vi "BRig_Host_dataRunState__entryAdd_v4.vi"(0 "input_dataPlot":u16[][](array[numeric]), 1 "input_dataTS":u16[][](array[numeric]), 2 "input_idx":i32[](array[numeric]), 4 "input_nTrial":u16, 5 "input_LorR":u16, 7 "input_sSelection":u16, 8 "input_trig_l2":u16, 9 "input_tSelection":u16, 10 "input_trig_l1":u16, 11 "input_tSelectionPlot":u16, 12 "input_DAB_flipLR":u16, 13 "input_iSelection":u16) -> (14 "output_dataPlot":u16[][](array[numeric]), 15 "output_dataTS":u16[][](array[numeric]), 16 "output_idx":i32[](array[numeric]), 18 "output_updatePlot":bool)   [LabVIEW 2014]
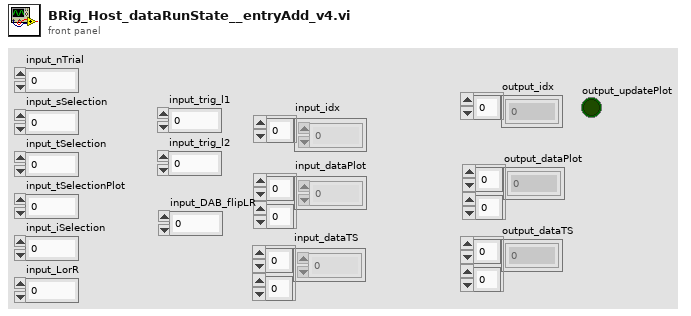
[diagram p1: front panel]
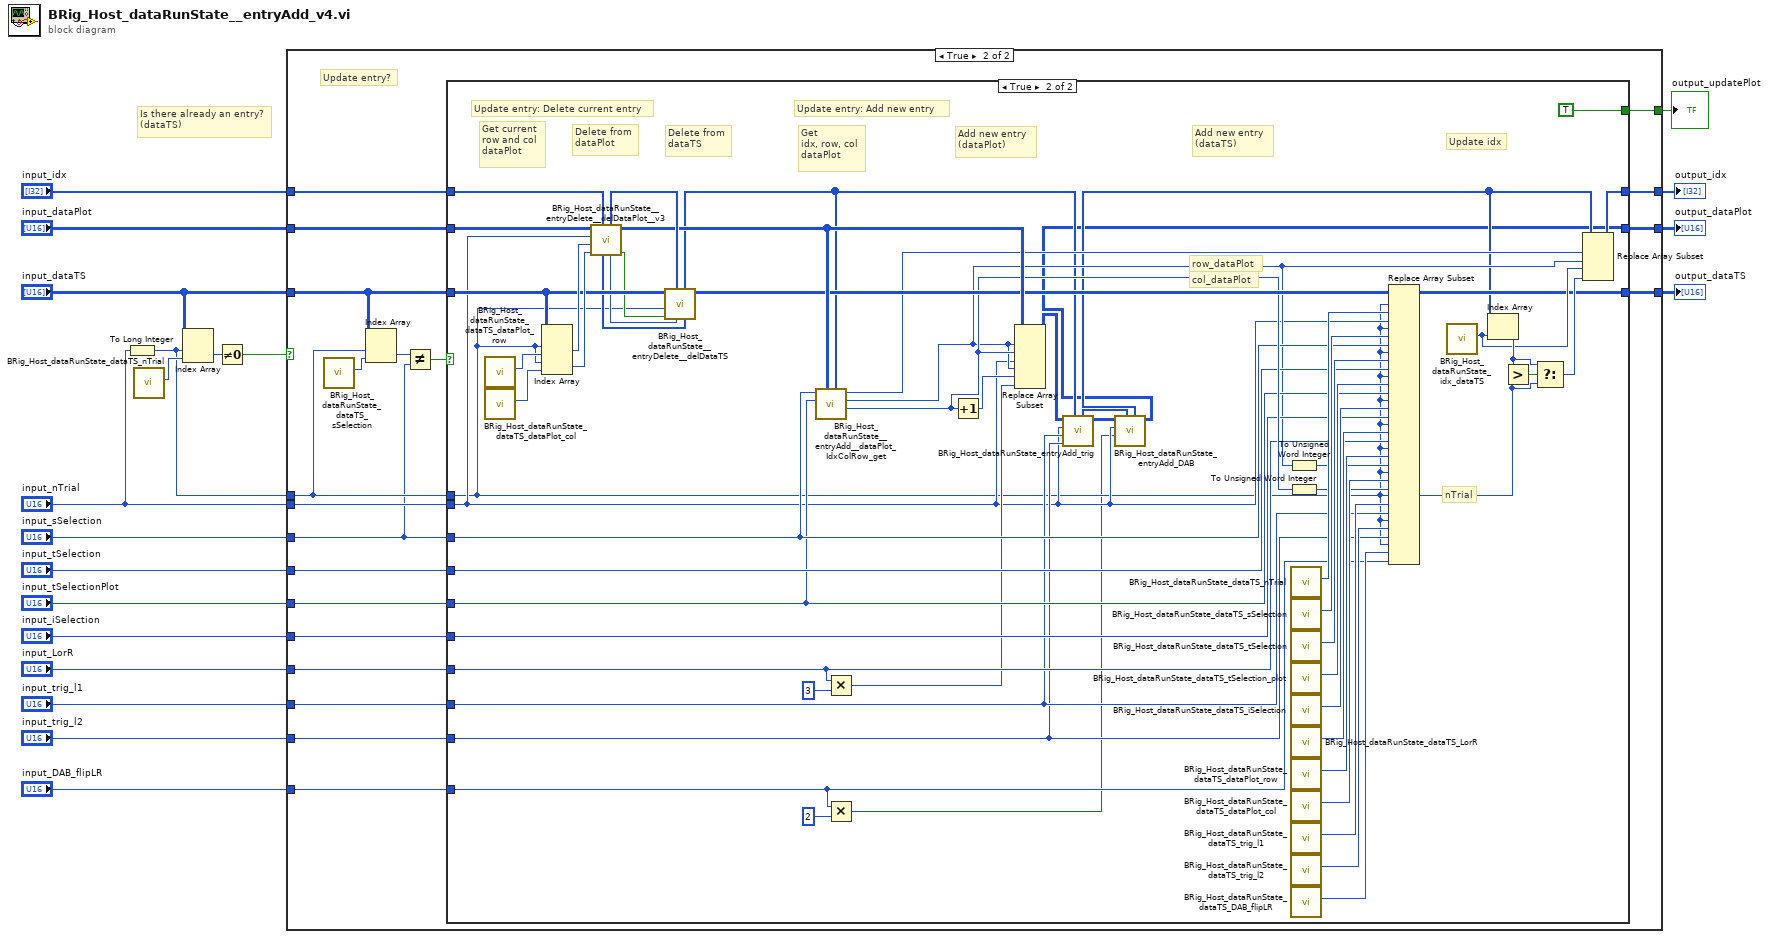
[diagram p0: block diagram]
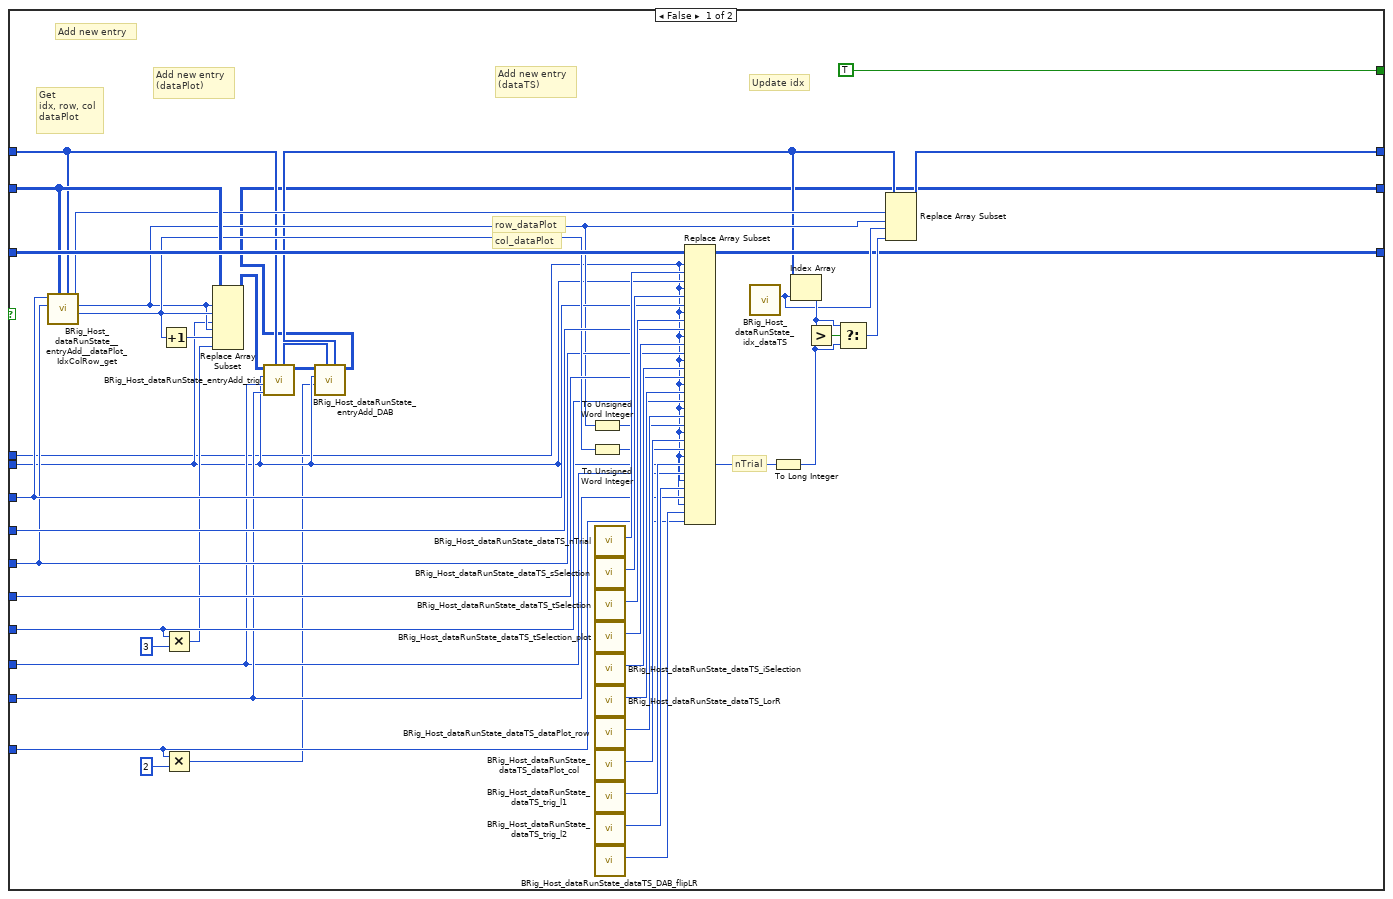
[diagram p2: hidden frame]
diagram:
  # "Is there already an entry?\n(dataTS)"
  n1 = To Long Integer(number="input_nTrial") -> (32bit integer=w16:i32)
  n2 = call "BRig_Host_dataRunState_dataTS_nTrial.vi"() -> ("output_idx_dataTS_nTrial"=w20:i32)  [unwired: 11 in]
  n3 = Index Array(array="input_dataTS", index (row)=w16, index (col)=w20) -> (element=w19:u16)
  n4 = Not Equal To 0?(x=w19) -> (x != 0?=w18:bool)
  n5 = case shown="True" w18 {
    tunnel: "input_nTrial" -> [w26 w77]
    tunnel: w16 -> [w25 w79]
    tunnel: "input_dataTS" -> [w67 w81]
    tunnel: "input_idx" -> [w33 w85]
    tunnel: "input_dataPlot" -> [w45 w83]
    tunnel: "input_sSelection" -> [w42 w71]
    tunnel: "input_tSelectionPlot" -> [w41 w78]
    tunnel: "input_iSelection" -> [w55 w74]
    tunnel: "input_LorR" -> [w36 w76]
    tunnel: [w57 w84] -> w7
    tunnel: [w27 w82] -> w6
    tunnel: [w50 w80] -> w5
    tunnel: "input_tSelection" -> [w56 w75]
    tunnel: [TRUE w73] -> w4
    tunnel: "input_trig_l1" -> [w31 w70]
    tunnel: "input_trig_l2" -> [w32 w69]
    tunnel: "input_DAB_flipLR" -> [w22 w68]
    frame False {
      # "Get\nidx, row, col\ndataPlot"
      # "nTrial"
      # "row_dataPlot"
      # "col_dataPlot"
      # "Update idx"
      # "Add new entry\n(dataPlot)"
      # "Add new entry"
      # "Add new entry\n(dataTS)"
      n6 = call "BRig_Host_dataRunState__entryAdd__dataPlot_IdxColRow_get.vi"("input_idx"=w33, "input_dataPlot"=w45, "input_tSelectionPlot"=w41, "input_sSelection"=w42) -> ("output_col_dataPlot"=w43:i32, "output_row_dataPlot"=w40:i32, "output_idx_dataPlot"=w44:i32)  [unwired: 5 in]
      n7 = Increment(x=w43) -> (x+1=w58:i32)
      n8 = Multiply(x=w36, y=u16 3) -> (x*y=w35:u16)
      n9 = Multiply(x=w22, y=u16 2) -> (x*y=w21:u16)
      n10 = Replace Array Subset(array=w45, new element #1=w26, index (row) #1=w40, index (col) #1=w43, new element #2=w35, index (row) #2=w40, index (col) #2=w58) -> (w34:u16[][])
      n11 = call "BRig_Host_dataRunState_entryAdd_trig.vi"("input_idx"=w33, "input_trig_l2"=w32, "input_trig_l1"=w31, "input_nTrial"=w26, "input_dataPlot"=w34) -> ("output_dataPlot"=w30:u16[][], "output_idx"=w28:i32[])  [unwired: 5 in]
      n12 = call "BRig_Host_dataRunState_entryAdd_DAB.vi"("input_idx"=w28, "input_DAB_flipLR"=w21, "input_nTrial"=w26, "input_dataPlot"=w30) -> ("output_dataPlot"=w27:u16[][], "output_idx"=w29:i32[])  [unwired: 6 in]
      n13 = To Unsigned Word Integer(number=w40) -> (unsigned 16bit integer=w49:u16)
      n14 = To Unsigned Word Integer(number=w43) -> (unsigned 16bit integer=w48:u16)
      n15 = call "BRig_Host_dataRunState_dataTS_nTrial.vi"() -> ("output_idx_dataTS_nTrial"=w66:i32)  [unwired: 11 in]
      n16 = call "BRig_Host_dataRunState_dataTS_sSelection.vi"() -> ("output_idx_dataTS_sSelection"=w65:i32)  [unwired: 11 in]
      n17 = call "BRig_Host_dataRunState_dataTS_tSelection.vi"() -> ("output_idx_dataTS_tSelection"=w64:i32)  [unwired: 11 in]
      n18 = call "BRig_Host_dataRunState_dataTS_tSelection_plot.vi"() -> ("output_idx_dataTS_tSelection_plot"=w63:i32)  [unwired: 11 in]
      n19 = call "BRig_Host_dataRunState_dataTS_iSelection.vi"() -> ("output_idx_dataTS_iSelection"=w62:i32)  [unwired: 11 in]
      n20 = call "BRig_Host_dataRunState_dataTS_LorR.vi"() -> ("output_idx_dataTS_LorR"=w61:i32)  [unwired: 11 in]
      n21 = call "BRig_Host_dataRunState_dataTS_dataPlot_row.vi"() -> ("output_idx_dataTS_dataPlot_row"=w60:i32)  [unwired: 11 in]
      n22 = call "BRig_Host_dataRunState_dataTS_dataPlot_col.vi"() -> ("output_idx_dataTS_dataPlot_col"=w59:i32)  [unwired: 11 in]
      n23 = call "BRig_Host_dataRunState_dataTS_trig_l1.vi"() -> ("output_idx_dataTS_trig_l1"=w38:i32)  [unwired: 11 in]
      n24 = call "BRig_Host_dataRunState_dataTS_trig_l2.vi"() -> ("output_idx_dataTS_trig_l2"=w37:i32)  [unwired: 11 in]
      n25 = call "BRig_Host_dataRunState_dataTS_DAB_flipLR.vi"() -> ("output_idx_dataTS_DAB_flipLR"=w24:i32)  [unwired: 11 in]
      n26 = Replace Array Subset(array=w67, new element #1=w26, index (row) #1=w25, index (col) #1=w66, new element #2=w42, index (row) #2=w25, index (col) #2=w65, new element #3=w56, index (row) #3=w25, index (col) #3=w64, new element #4=w41, index (row) #4=w25, index (col) #4=w63, new element #5=w55, index (row) #5=w25, index (col) #5=w62, new element #6=w36, index (row) #6=w25, index (col) #6=w61, new element #7=w49, index (row) #7=w25, index (col) #7=w60, new element #8=w48, index (row) #8=w25, index (col) #8=w59, new element #9=w31, index (row) #9=w25, index (col) #9=w38, new element #10=w32, index (row) #10=w25, index (col) #10=w37, new element #11=w22, index (row) #11=w25, index (col) #11=w24) -> (w50:u16[][])
      n27 = call "BRig_Host_dataRunState_idx_dataTS.vi"() -> ("output_idx_dataTS"=w52:i32)  [unwired: 11 in]
      n28 = To Long Integer(number=w26) -> (32bit integer=w47:i32)
      n29 = Index Array(array=w29, index=w52) -> (element=w53:i32)
      n30 = Greater?(x=w53, y=w47) -> (0:w54:bool)
      n31 = Select(t=w53, s=w54, f=w47) -> (s? t:f=w51:i32)
      n32 = Replace Array Subset(array=w29, new element #1=w40, index #1=w44, new element #2=w51, index #2=w52) -> (w57:i32[])
    }
    frame True {
      # "Update entry?"
      n33 = call "BRig_Host_dataRunState_dataTS_sSelection.vi"() -> ("output_idx_dataTS_sSelection"=w72:i32)  [unwired: 11 in]
      n34 = Index Array(array=w81, index (row)=w79, index (col)=w72) -> (element=w87:u16)
      n35 = Not Equal?(x=w87, y=w71) -> (x != y?=w86:bool)
      n36 = case shown="True" w86 {
        tunnel: w85 -> [w90 w142]
        tunnel: [w90 w121] -> w84
        tunnel: w83 -> [w89 w145]
        tunnel: [w89 w97] -> w82
        tunnel: w81 -> [w88 w141]
        tunnel: [w88 w118] -> w80
        tunnel: w79 -> [_ w95]
        tunnel: w71 -> [_ w115]
        tunnel: w78 -> [_ w113]
        tunnel: w77 -> [_ w96]
        tunnel: w76 -> [_ w106]
        tunnel: w75 -> [_ w114]
        tunnel: w74 -> [_ w112]
        tunnel: [_ TRUE] -> w73
        tunnel: w70 -> [_ w103]
        tunnel: w69 -> [_ w102]
        tunnel: w68 -> [_ w92]
        frame False {
          # "Do nothing"
        }
        frame True {
          # "nTrial"
          # "row_dataPlot"
          # "col_dataPlot"
          # "Update idx"
          # "Add new entry\n(dataPlot)"
          # "Add new entry\n(dataTS)"
          # "Get\nidx, row, col\ndataPlot"
          # "Update entry: Add new entry"
          # "Delete from\ndataTS"
          # "Delete from\ndataPlot"
          # "Get current\nrow and col\ndataPlot"
          # "Update entry: Delete current entry"
          n37 = call "BRig_Host_dataRunState_dataTS_dataPlot_row.vi"() -> ("output_idx_dataTS_dataPlot_row"=w147:i32)  [unwired: 11 in]
          n38 = call "BRig_Host_dataRunState_dataTS_dataPlot_col.vi"() -> ("output_idx_dataTS_dataPlot_col"=w146:i32)  [unwired: 11 in]
          n39 = Index Array(array=w141, index (row) #1=w95, index (col) #1=w147, index (row) #2=w95, index (col) #2=w146) -> (element #1=w143:u16, element #2=w144:u16)
          n40 = call "BRig_Host_dataRunState__entryDelete__delDataPlot__v3.vi"("input_idx"=w142, "input_col_dataPlot"=w144, "input_row_dataPlot"=w143, "input_nTrial"=w96, "input_dataPlot"=w145) -> (0:"output_arrTrials"=w139:bool, "output_dataPlot"=w120:u16[][], "output_arrTrials_length"=w138:i32, "output_idx"=w140:i32[], 6:"output_arrTrials"=w137:i32[])  [unwired: 2 in]
          n41 = call "BRig_Host_dataRunState__entryDelete__delDataTS.vi"(4:"output_arrTrials"=w137, "output_arrTrials_length"=w138, "input_idx"=w140, 8:"output_arrTrials"=w139, "input_nTrial"=w95, "input_dataTS"=w141) -> ("output_dataTS"=w119:u16[][], "output_idx"=w101:i32[])  [unwired: 4 in]
          n42 = call "BRig_Host_dataRunState__entryAdd__dataPlot_IdxColRow_get.vi"("input_idx"=w101, "input_dataPlot"=w120, "input_tSelectionPlot"=w113, "input_sSelection"=w115) -> ("output_col_dataPlot"=w116:i32, "output_row_dataPlot"=w110:i32, "output_idx_dataPlot"=w117:i32)  [unwired: 5 in]
          n43 = Multiply(x=w106, y=u16 3) -> (x*y=w105:u16)
          n44 = Multiply(x=w92, y=u16 2) -> (x*y=w91:u16)
          n45 = Increment(x=w116) -> (x+1=w128:i32)
          n46 = Replace Array Subset(array=w120, new element #1=w96, index (row) #1=w110, index (col) #1=w116, new element #2=w105, index (row) #2=w110, index (col) #2=w128) -> (w104:u16[][])
          n47 = call "BRig_Host_dataRunState_entryAdd_trig.vi"("input_idx"=w101, "input_trig_l2"=w102, "input_trig_l1"=w103, "input_nTrial"=w96, "input_dataPlot"=w104) -> ("output_dataPlot"=w100:u16[][], "output_idx"=w98:i32[])  [unwired: 5 in]
          n48 = call "BRig_Host_dataRunState_entryAdd_DAB.vi"("input_idx"=w98, "input_DAB_flipLR"=w91, "input_nTrial"=w96, "input_dataPlot"=w100) -> ("output_dataPlot"=w97:u16[][], "output_idx"=w99:i32[])  [unwired: 6 in]
          n49 = To Unsigned Word Integer(number=w110) -> (unsigned 16bit integer=w123:u16)
          n50 = To Unsigned Word Integer(number=w116) -> (unsigned 16bit integer=w122:u16)
          n51 = call "BRig_Host_dataRunState_dataTS_nTrial.vi"() -> ("output_idx_dataTS_nTrial"=w136:i32)  [unwired: 11 in]
          n52 = call "BRig_Host_dataRunState_dataTS_sSelection.vi"() -> ("output_idx_dataTS_sSelection"=w135:i32)  [unwired: 11 in]
          n53 = call "BRig_Host_dataRunState_dataTS_tSelection.vi"() -> ("output_idx_dataTS_tSelection"=w134:i32)  [unwired: 11 in]
          n54 = call "BRig_Host_dataRunState_dataTS_tSelection_plot.vi"() -> ("output_idx_dataTS_tSelection_plot"=w133:i32)  [unwired: 11 in]
          n55 = call "BRig_Host_dataRunState_dataTS_iSelection.vi"() -> ("output_idx_dataTS_iSelection"=w132:i32)  [unwired: 11 in]
          n56 = call "BRig_Host_dataRunState_dataTS_LorR.vi"() -> ("output_idx_dataTS_LorR"=w131:i32)  [unwired: 11 in]
          n57 = call "BRig_Host_dataRunState_dataTS_dataPlot_row.vi"() -> ("output_idx_dataTS_dataPlot_row"=w130:i32)  [unwired: 11 in]
          n58 = call "BRig_Host_dataRunState_dataTS_dataPlot_col.vi"() -> ("output_idx_dataTS_dataPlot_col"=w129:i32)  [unwired: 11 in]
          n59 = call "BRig_Host_dataRunState_dataTS_trig_l1.vi"() -> ("output_idx_dataTS_trig_l1"=w109:i32)  [unwired: 11 in]
          n60 = call "BRig_Host_dataRunState_dataTS_trig_l2.vi"() -> ("output_idx_dataTS_trig_l2"=w108:i32)  [unwired: 11 in]
          n61 = call "BRig_Host_dataRunState_dataTS_DAB_flipLR.vi"() -> ("output_idx_dataTS_DAB_flipLR"=w94:i32)  [unwired: 11 in]
          n62 = Replace Array Subset(array=w119, new element #1=w96, index (row) #1=w95, index (col) #1=w136, new element #2=w115, index (row) #2=w95, index (col) #2=w135, new element #3=w114, index (row) #3=w95, index (col) #3=w134, new element #4=w113, index (row) #4=w95, index (col) #4=w133, new element #5=w112, index (row) #5=w95, index (col) #5=w132, new element #6=w106, index (row) #6=w95, index (col) #6=w131, new element #7=w123, index (row) #7=w95, index (col) #7=w130, new element #8=w122, index (row) #8=w95, index (col) #8=w129, new element #9=w103, index (row) #9=w95, index (col) #9=w109, new element #10=w102, index (row) #10=w95, index (col) #10=w108, new element #11=w92, index (row) #11=w95, index (col) #11=w94) -> (w118:u16[][])
          n63 = call "BRig_Host_dataRunState_idx_dataTS.vi"() -> ("output_idx_dataTS"=w125:i32)  [unwired: 11 in]
          n64 = Index Array(array=w99, index=w125) -> (element=w126:i32)
          n65 = Greater?(x=w126, y=w95) -> (0:w127:bool)
          n66 = Select(t=w126, s=w127, f=w95) -> (s? t:f=w124:i32)
          n67 = Replace Array Subset(array=w99, new element #1=w110, index #1=w117, new element #2=w124, index #2=w125) -> (w121:i32[])
        }
      }
    }
  }
  "output_idx" <- w7
  "output_dataPlot" <- w6
  "output_dataTS" <- w5
  "output_updatePlot" <- w4
